vi "Wärmepumpe.GenLookUpHeizleistung.vi"(0 "Wärmepumpe in":refnum<data-value>, 5 "Error in":errorcluster) -> (14 "Wärmepumpe out":refnum<data-value>, 19 "Error out":errorcluster)   [LabVIEW 2016, in "Wärmepumpe.lvclass"]
uses:
  <vilib>/Analysis/1siggen.llb/Ramp Pattern by Samples.vi
  <vilib>/gmath/interp.llb/Create Mesh Grid (2D) (x,y arrays).vi
  <vilib>/gmath/interp.llb/Interpolate 2D Scattered (2D).vi
  <vilib>/gmath/NI_AAL_Interpolation.lvlib
  <vilib>/gmath/NI_Gmath.lvlib
  <vilib>/Analysis/NI_AALBase.lvlib
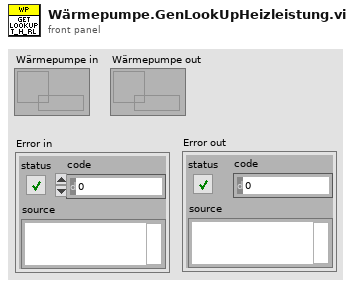
[diagram p1: front panel]
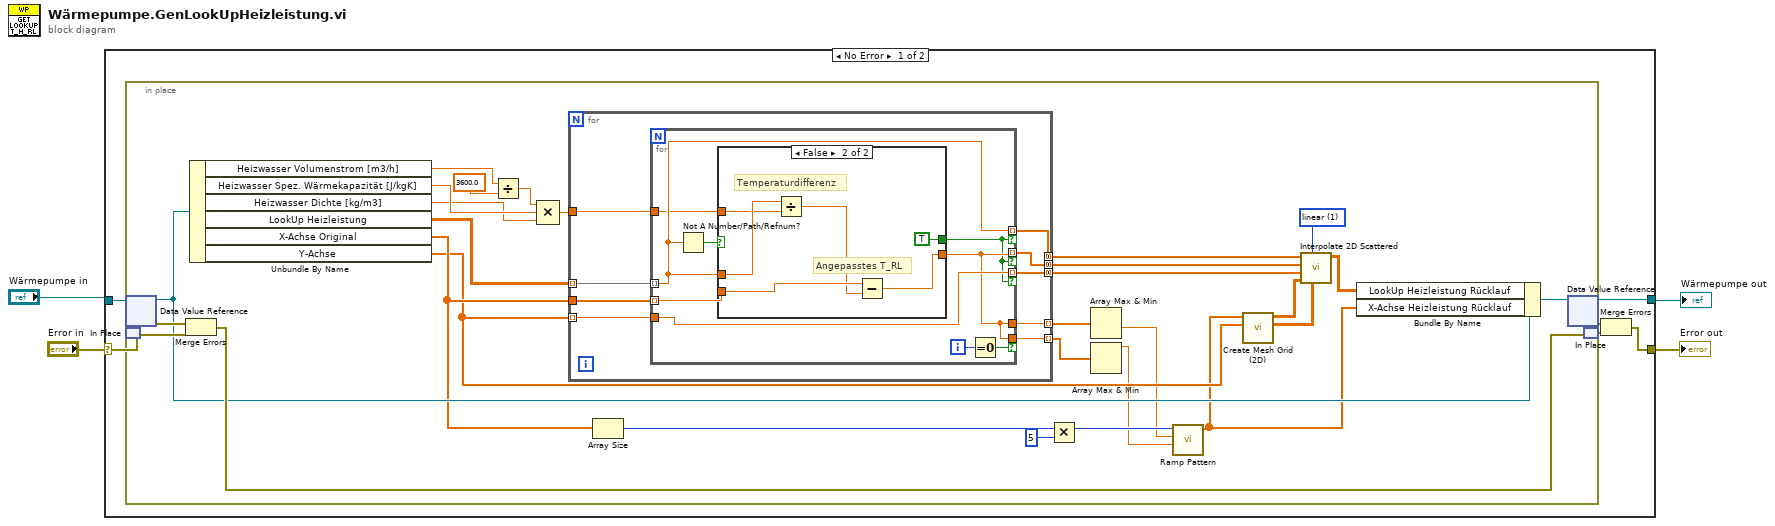
[diagram p0: block diagram]
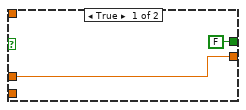
[diagram p2: hidden frame]
diagram:
  n1 = case shown="No Error" "Error in" {
    selector: "Error in" -> [w8 w67]
    tunnel: [w7 w66] -> w3
    tunnel: [w6 w67] -> w2
    tunnel: "Wärmepumpe in" -> [w5 w66]
    frame No Error {
      n2 = in-place {
        w24 = 1 items=["nearest", "linear", "cubic", "biharmonic spline "] ("method")
        n3 = in-place-dvr #1(w5) -> (w35:refnum<class "Wärmepumpe.lvclass">, w39:errorcluster)
        n4 = in-place-match #2(w8) -> (w38:errorcluster)
        n5 = Merge Errors(w39, w38) -> (w37:errorcluster)
        n6 = Unbundle By Name(w35) -> ("Heizwasser Volumenstrom [m3/h]"=w14:dbl, "Heizwasser Spez. Wärmekapazität [J/kgK]"=w12:dbl, "Heizwasser Dichte [kg/m3]"=w11:dbl, "LookUp Heizleistung"=w34:dbl[][], "X-Achse Original"=w28:dbl[], "Y-Achse"=w23:dbl[])
        n7 = Divide(x=w14, y=3600.0) -> (x/y=w13:dbl)
        n8 = Compound Arithmetic op=MULTIPLY(w13, w12, w11) -> (w16:dbl)
        n9 = for {
          tunnel: w34 -> [w48] mode=indexing
          tunnel: w28 -> [w47]
          tunnel: w23 -> [w46] mode=indexing
          tunnel: [w45] -> w33 mode=concatenating
          tunnel: [w44] -> w29 mode=concatenating
          tunnel: [w43] -> w32 mode=concatenating
          tunnel: [w42] -> w20 mode=indexing
          tunnel: [w41] -> w18 mode=indexing
          tunnel: w16 -> [w40]
          n10 = for {
            tunnel: w48 -> [w52] mode=indexing
            tunnel: w47 -> [w57] mode=indexing
            tunnel: w46 -> [w56]
            tunnel: [w52] -> w45 mode=indexing if=w50
            tunnel: [w54] -> w44 mode=indexing if=w50
            tunnel: [w56] -> w43 mode=indexing if=w50
            tunnel: [w54] -> w42
            tunnel: [w54] -> w41 if=w53
            tunnel: w40 -> [w49]
            i -> [w55]
            n11 = Not A Number/Path/Refnum?(number/path/refnum=w52) -> (NaN/Path/Refnum?=w51:bool)
            n12 = case shown="False" w51 {
              tunnel: w57 -> [_ w65]
              tunnel: w52 -> [w59 w63]
              tunnel: [w59 w62] -> w54
              tunnel: [FALSE TRUE] -> w50
              tunnel: w49 -> [_ w60]
              frame True {
              }
              frame False {
                # "Angepasstes T_RL"
                # "Temperaturdifferenz"
                n13 = Divide(x=w63, y=w60) -> (x/y=w64:dbl)
                n14 = Subtract(x=w65, y=w64) -> (x-y=w62:dbl)
              }
            }
            n15 = Equal To 0?(x=w55) -> (x = 0?=w53:bool)
          }
        }
        n16 = Array Size(array=w28) -> (size(s)=w27:i32)
        n17 = Multiply(x=w27, y=5) -> (x*y=w26:i32)
        n18 = Array Max & Min(array=w20) -> (min value=w19:dbl)  [unwired: 3 out]
        n19 = Array Max & Min(array=w18) -> (max value=w17:dbl)  [unwired: 3 out]
        n20 = call-poly <vilib>:"Ramp Pattern.vi"("start"=w17, "end"=w19, "samples"=w26) -> ("Ramp Pattern"=w22:dbl[])  [unwired: 7 in, 1 out]
        n21 = call-poly <vilib>:"Create Mesh Grid (2D).vi"("y domain"=w23, "x domain"=w22) -> ("Y"=w30:dbl[][], "X"=w31:dbl[][])  [unwired: 7 in, 1 out]
        n22 = call-poly <vilib>:"Interpolate 2D Scattered.vi"("Yi"=w30, "method"=w24, "Xi"=w31, "Y"=w32, "X"=w29, "Z"=w33) -> ("Zi"=w21:dbl[][])  [unwired: 4 in, 1 out]
        n23 = Bundle By Name(cluster=w35, "LookUp Heizleistung Rücklauf"=w21, "X-Achse Heizleistung Rücklauf"=w22) -> (w36:refnum<class "Wärmepumpe.lvclass">)
        n24 = in-place-dvr #1(w36) -> (w7:refnum<data-value>, w10:errorcluster)
        n25 = in-place-match #2(w37) -> (w9:errorcluster)
      }
      n26 = Merge Errors(w10, w9) -> (w6:errorcluster)
    }
    frame Error {
    }
  }
  "Wärmepumpe out" <- w3
  "Error out" <- w2
